vi "bintodeci.vi"(11 "Binary number":i32=422 format="%.0b") -> (3 "Decimal number":u8)   [LabVIEW 2013]
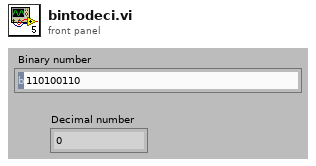
[diagram p1: front panel]
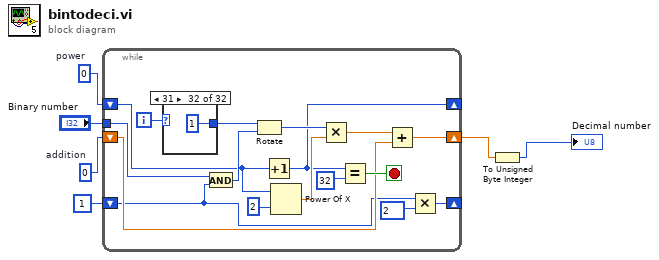
[diagram p0: block diagram]
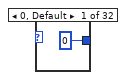
[diagram p2: hidden frame]
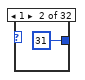
[diagram p3: hidden frame]
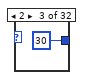
[diagram p4: hidden frame]
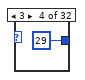
[diagram p5: hidden frame]
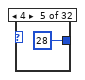
[diagram p6: hidden frame]
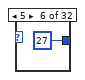
[diagram p7: hidden frame]
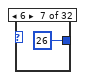
[diagram p8: hidden frame]
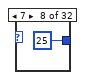
[diagram p9: hidden frame]
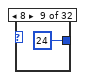
[diagram p10: hidden frame]
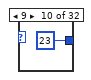
[diagram p11: hidden frame]
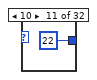
[diagram p12: hidden frame]
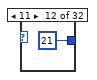
[diagram p13: hidden frame]
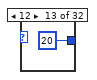
[diagram p14: hidden frame]
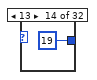
[diagram p15: hidden frame]
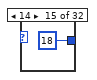
[diagram p16: hidden frame]
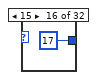
[diagram p17: hidden frame]
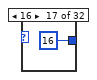
[diagram p18: hidden frame]
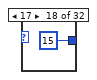
[diagram p19: hidden frame]
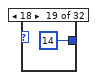
[diagram p20: hidden frame]
diagram:
  w5 = i16 0  # addition
  w6 = 0  # power
  n1 = while {
    shift-right: [w12] -> _
    shift-left: w6 -> [w20]
    shift-right: [w15] -> w2
    shift-left: w5 -> [w18]
    tunnel: "Binary number" -> [w10]
    shift-right: [w7] -> _
    shift-left: 1 ("x") -> [w9]
    i -> [w13]
    stop <- w19 stop-if-true
    n2 = case shown="31" w13 {
      tunnel: [0 31 30 29 28 27 26 25 24 23 22 21 20 19 18 17 16 15 14 13 12 11 10 9 8 7 6 5 4 3 2 1] -> w14
      frame 0, Default {
      }
      frame 1 {
      }
      frame 2 {
      }
      frame 3 {
      }
      frame 4 {
      }
      frame 5 {
      }
      frame 6 {
      }
      frame 7 {
      }
      frame 8 {
      }
      frame 9 {
      }
      frame 10 {
      }
      frame 11 {
      }
      frame 12 {
      }
      frame 13 {
      }
      frame 14 {
      }
      frame 15 {
      }
      frame 16 {
      }
      frame 17 {
      }
      frame 18 {
      }
      frame 19 {
      }
      frame 20 {
      }
      frame 21 {
      }
      frame 22 {
      }
      frame 23 {
      }
      frame 24 {
      }
      frame 25 {
      }
      frame 26 {
      }
      frame 27 {
      }
      frame 28 {
      }
      frame 29 {
      }
      frame 30 {
      }
      frame 31 {
      }
    }
    n3 = And(x=w10, y=w9) -> (x .and. y?=w23:i32)
    n4 = Rotate(1:w23, 2:w14) -> (0:w21:i32)
    n5 = Increment(x=w20) -> (x+1=w12:i32)
    n6 = Power Of X(1:2 ("x"), 2:w20) -> (0:w17:dbl)
    n7 = Multiply(x=w21, y=w17) -> (x*y=w16:dbl)
    n8 = Equal?(x=w12, y=32) -> (x = y?=w19:bool)
    n9 = Add(x=w16, y=w18) -> (x+y=w15:dbl)
    n10 = Multiply(x=w9, y=2) -> (x*y=w7:i32)
  }
  n11 = To Unsigned Byte Integer(number=w2) -> (unsigned 8bit integer=→"Decimal number":u8)
